vi "2048.vi"() -> ()   [LabVIEW 2013]
uses:
  <vilib>/Utility/file.llb/Read From Spreadsheet File (DBL).vi
  <vilib>/Utility/file.llb/Write To Spreadsheet File (I64).vi
panel:
  out "分数":i64=3
  in  "清空按钮":bool
  in  "按钮（退出程序）":bool
  out "错误输出":errorcluster
  in  "错误输入":errorcluster caption="错误输入（无错误）"
  out "2048":u16[][](array[ring])
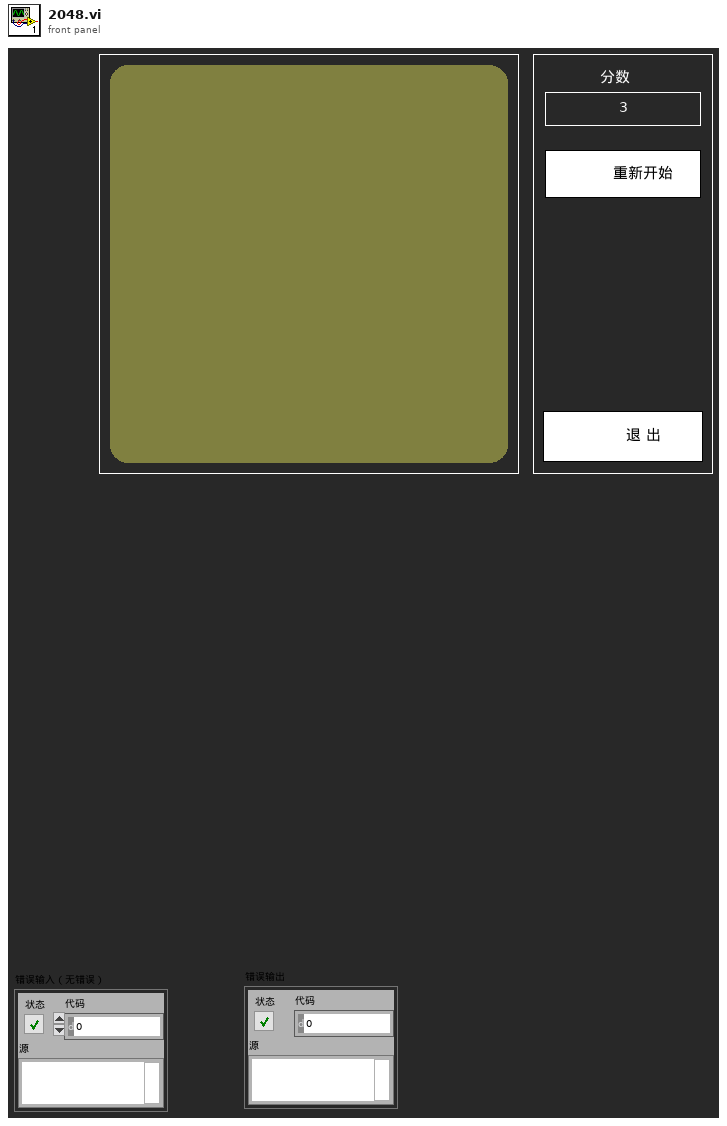
[diagram p1: front panel]
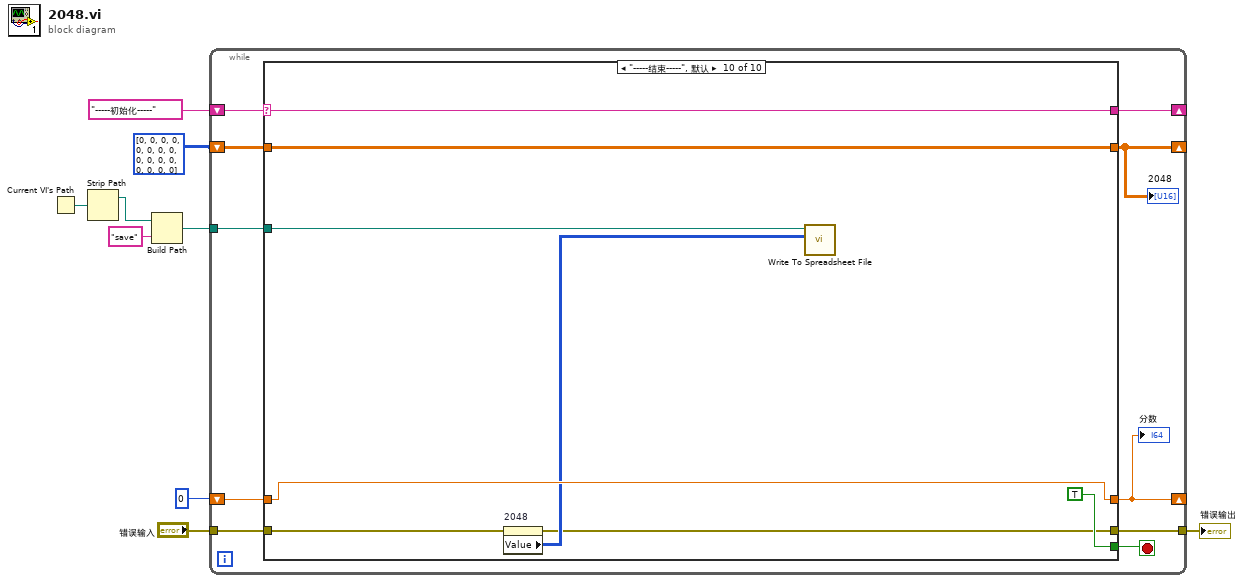
[diagram p0: block diagram]
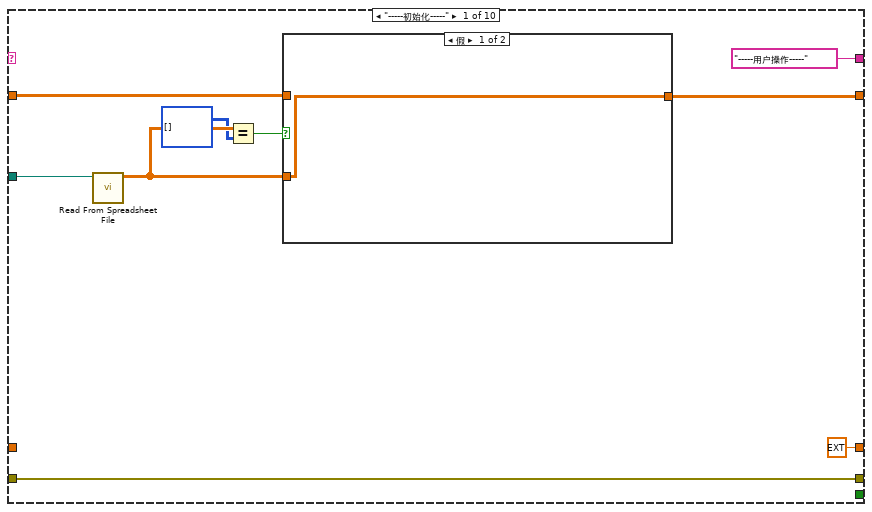
[diagram p2: hidden frame]
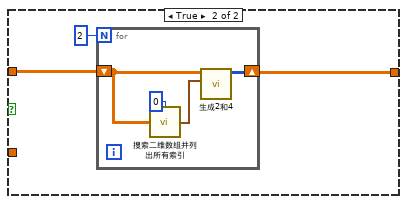
[diagram p3: hidden frame]
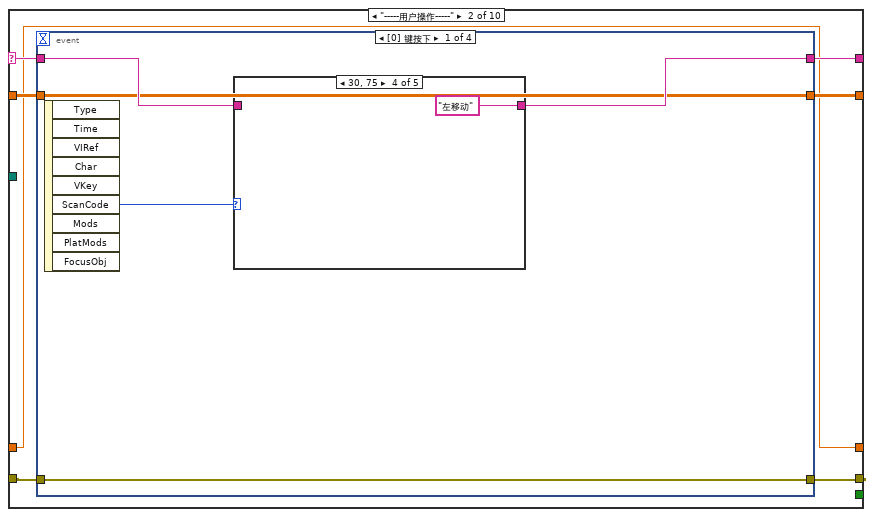
[diagram p4: hidden frame]
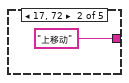
[diagram p6: hidden frame]
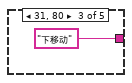
[diagram p7: hidden frame]
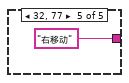
[diagram p8: hidden frame]
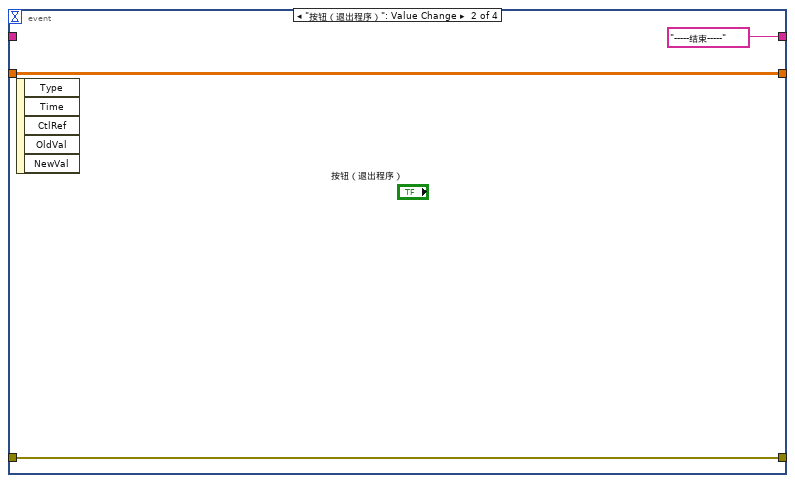
[diagram p9: hidden frame]
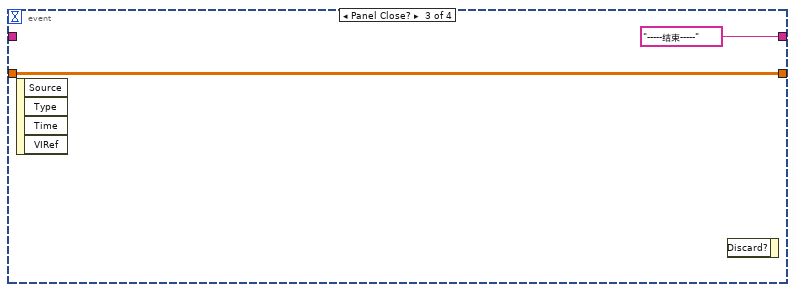
[diagram p10: hidden frame]
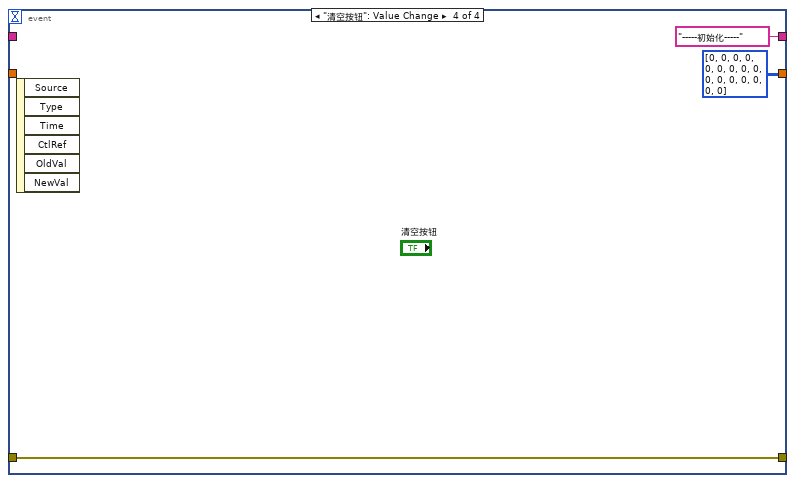
[diagram p11: hidden frame]
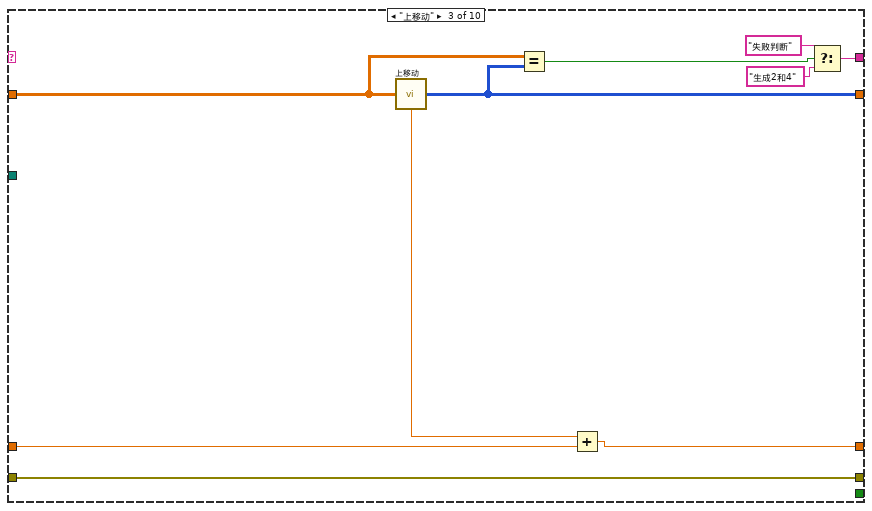
[diagram p12: hidden frame]
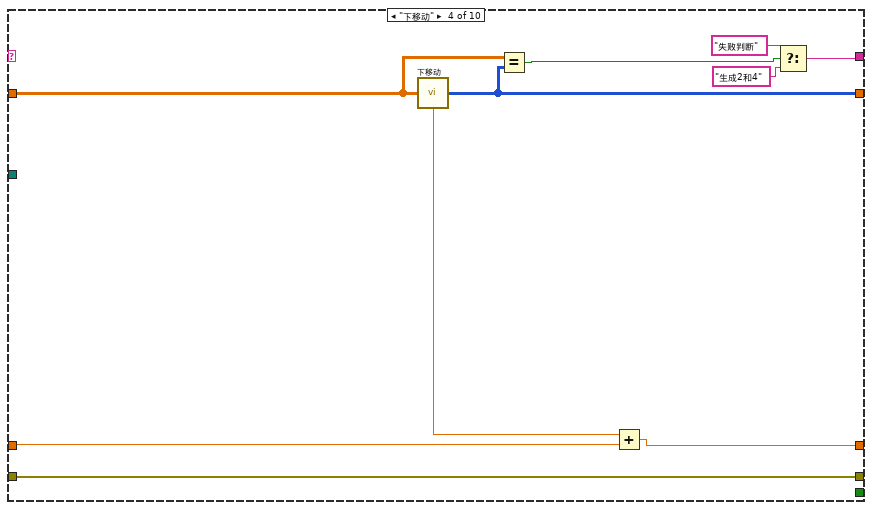
[diagram p13: hidden frame]
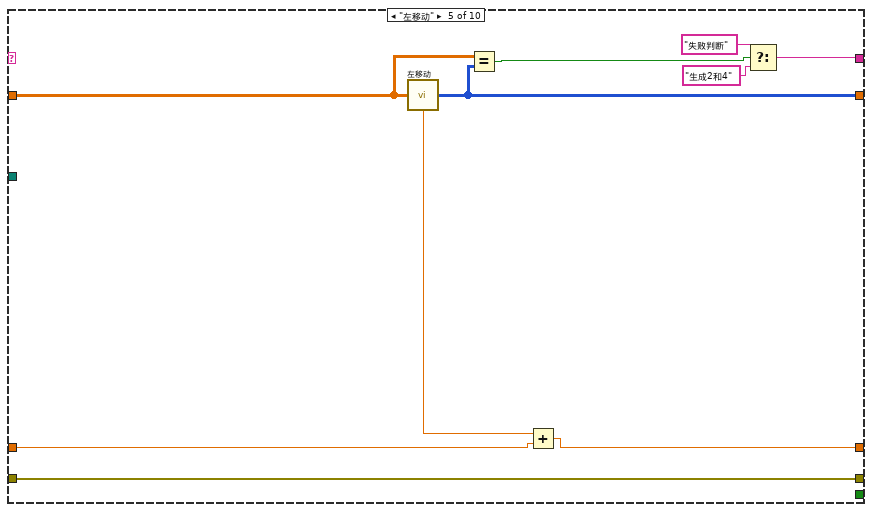
[diagram p14: hidden frame]
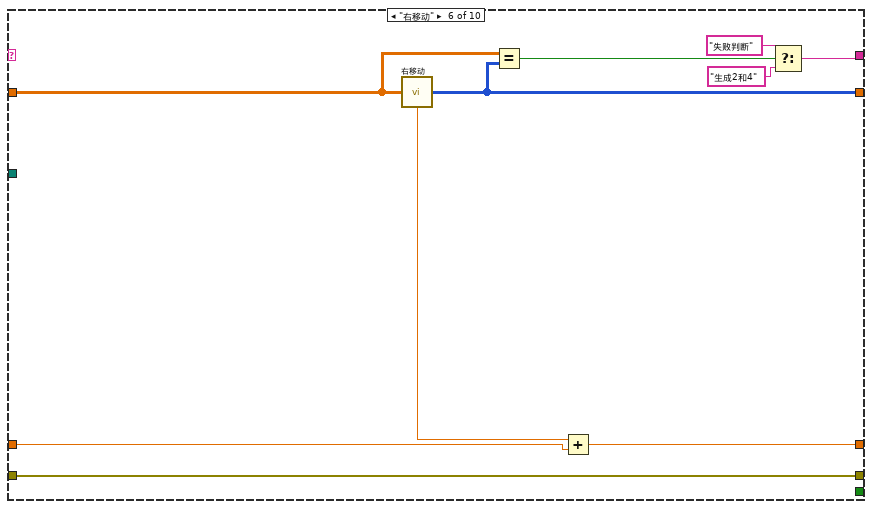
[diagram p15: hidden frame]
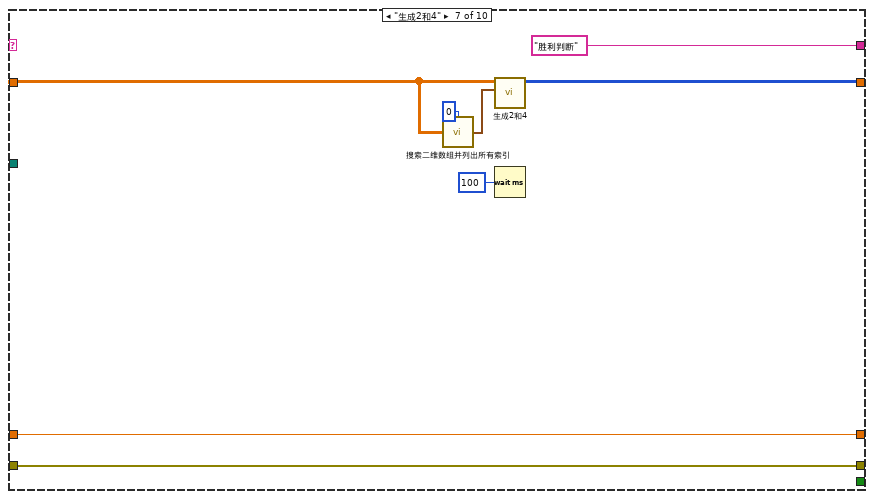
[diagram p16: hidden frame]
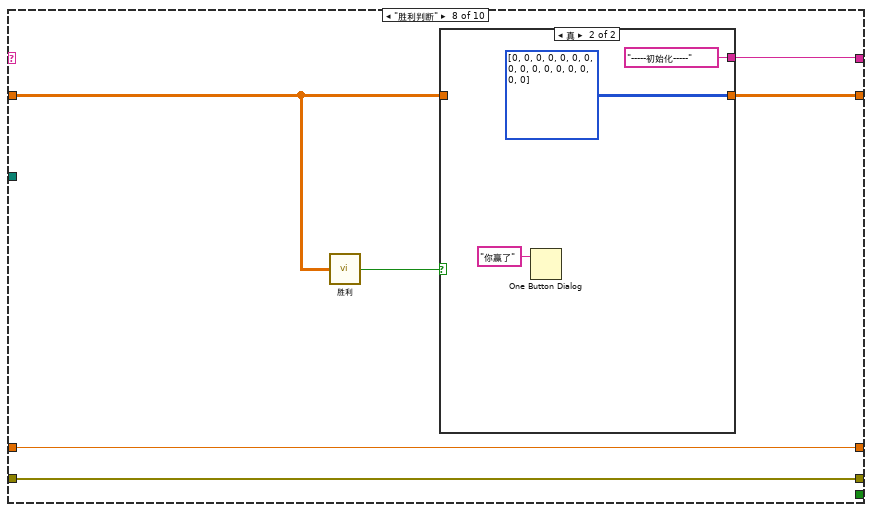
[diagram p17: hidden frame]
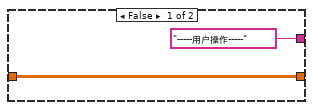
[diagram p18: hidden frame]
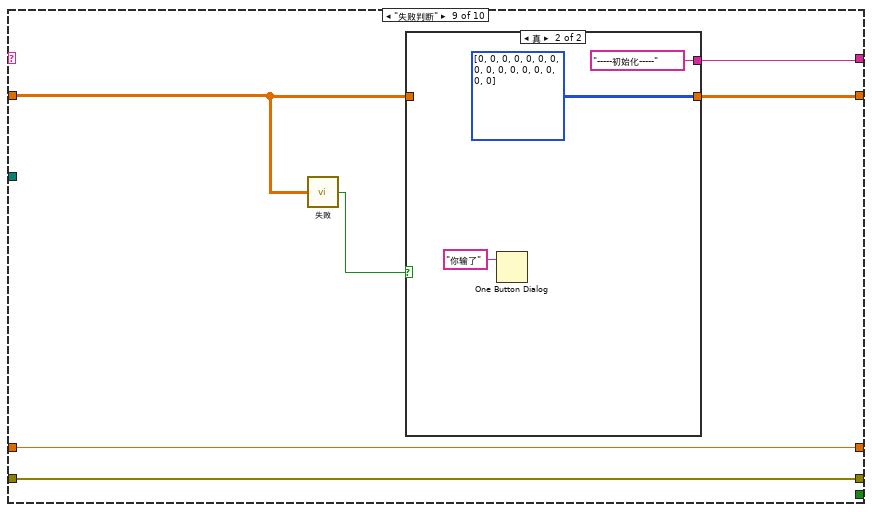
[diagram p19: hidden frame]
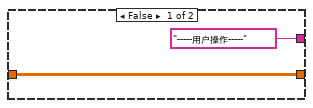
[diagram p20: hidden frame]
diagram:
  n1 = Current VI's Path() -> (path=w4:path)
  n2 = Strip Path(path=w4) -> (stripped path=w3:path)  [unwired: 1 out]
  n3 = Build Path(base path=w3, name or relative path="save" ("名称或相对路径")) -> (appended path=w1:path)
  n4 = while {
    shift-right: [w16] -> _
    shift-left: "-----初始化-----" -> [w17]
    tunnel: [w19] -> w8
    tunnel: "错误输入" -> [w18]
    shift-right: [w13] -> _
    shift-left: i32[][] [[0, 0, 0, 0], [0, 0, 0, 0], [0, 0, 0, 0], [0, 0, 0, 0]] ("2048") -> [w14]
    shift-right: [w11] -> _
    shift-left: 0 -> [w12]
    tunnel: w1 -> [w10]
    stop <- w15 stop-if-true
    n5 = case shown="\"-----结束-----\", 默认" w17 {
      selector: w17 -> [_ w40 _ _ _ _ _ _ _ w139]
      tunnel: [w23 w43 w71 w81 w91 w101 w109 w115 w126 w132] -> w19
      tunnel: w18 -> [w23 w42 w71 w81 w91 w101 w109 w115 w126 w133]
      tunnel: ["-----用户操作-----" w41 w68 w77 w87 w97 "胜利判断" w111 w125 w139] -> w16
      tunnel: [_ _ _ _ _ _ _ _ _ TRUE] -> w15
      tunnel: [w26 w39 w66 w76 w86 w96 w106 w113 w124 w137] -> w13
      tunnel: w14 -> [w27 w38 w67 w75 w85 w95 w105 w112 w123 w137]
      tunnel: w12 -> [_ w37 w63 w73 w83 w93 w102 w110 w121 w136]
      tunnel: [ext 0.0 w37 w62 w74 w82 w94 w102 w110 w121 w136] -> w11
      tunnel: w10 -> [w24 _ _ _ _ _ _ _ _ w135]
      frame "-----初始化-----" {
        n6 = call-poly <vilib>:"Read From Spreadsheet File.vi"("file path (dialog if empty)"=w24) -> ("all rows"=w21:dbl[][])  [unwired: 6 in, 4 out]
        n7 = Equal?(x=w21, y=i32[][] [] ("2048")) -> (x = y?=w22:bool)
        n8 = case shown="假" w22 {
          tunnel: w27 -> [_ w32]
          tunnel: [w29 w31] -> w26
          tunnel: w21 -> [w29 _]
          frame False {
          }
          frame True {
            n9 = for {
              N: 2 -> [_]
              shift-right: [w33] -> w31
              shift-left: w32 -> [w35]
              n10 = call "搜索二维数组并列出所有索引.vi"("搜索值"=0, "数组"=w35) -> ("索引数组"=w34:cluster{i32, i32}[])  [unwired: 2 in]
              n11 = call "生成2和4.vi"("索引数组"=w34, "2048输入"=w35) -> ("2048输出"=w33:i32[][])  [unwired: 9 in]
            }
          }
        }
      }
      frame "-----用户操作-----" {
        n12 = event shown="[0] 键按下" {
          selector: _ -> [_ _ _ _]
          dyn-events: _ -> [_ _ _ _]
          timeout: _ -> [_ _ _ _]
          tunnel: [w48 w56 _ w61] -> w43
          tunnel: w42 -> [w48 w56 _ w61]
          tunnel: [w47 "-----结束-----" "-----结束-----" "-----初始化-----"] -> w41
          tunnel: w40 -> [w46 _ _ _]
          tunnel: [w44 w54 w57 i32[][] [[0, 0, 0, 0], [0, 0, 0, 0], [0, 0, 0, 0], [0, 0, 0, 0]] ("2048")] -> w39
          tunnel: w38 -> [w44 w54 w57 _]
          event Key Down {
            n13 = event-data() -> ("ScanCode"=w45:i16)  [unwired: 1 in, 8 out]
            n14 = case shown="30, 75" w45 {
              tunnel: [w49 "上移动" "下移动" "左移动" "右移动"] -> w47
              tunnel: w46 -> [w49 _ _ _ _]
              frame 0, Default {
              }
              frame 17, 72 {
              }
              frame 31, 80 {
              }
              frame 30, 75 {
              }
              frame 32, 77 {
              }
            }
          }
          event "按钮（退出程序）": Value Change {
            n15 = event-data() -> ()  [unwired: 1 in, 5 out]
          }
          event Panel Close? {
            n16 = event-data() -> ()  [unwired: 1 in, 4 out]
            n17 = event-data() -> ()  [unwired: 2 in, 1 out]
          }
          event "清空按钮": Value Change {
            n18 = event-data() -> ()  [unwired: 1 in, 6 out]
          }
        }
      }
      frame "上移动" {
        n19 = call "上移动.vi"("移动前"=w67) -> ("移动后"=w66:i32[][], "分数"=w64:ext)  [unwired: 2 in]
        n20 = Equal?(x=w67, y=w66) -> (x = y?=w65:bool)
        n21 = Add(x=w64, y=w63) -> (x+y=w62:ext)
        n22 = Select(t="失败判断", s=w65, f="生成2和4") -> (s? t:f=w68:string)
      }
      frame "下移动" {
        n23 = call "下移动.vi"("移动前"=w75) -> ("移动后"=w76:i32[][], "分数"=w72:ext)  [unwired: 2 in]
        n24 = Equal?(x=w75, y=w76) -> (x = y?=w78:bool)
        n25 = Add(x=w72, y=w73) -> (x+y=w74:ext)
        n26 = Select(t="失败判断", s=w78, f="生成2和4") -> (s? t:f=w77:string)
      }
      frame "左移动" {
        n27 = call "左移动.vi"("移动前"=w85) -> ("移动后"=w86:i32[][], "分数"=w84:ext)  [unwired: 2 in]
        n28 = Equal?(x=w85, y=w86) -> (x = y?=w88:bool)
        n29 = Add(x=w84, y=w83) -> (x+y=w82:ext)
        n30 = Select(t="失败判断", s=w88, f="生成2和4") -> (s? t:f=w87:string)
      }
      frame "右移动" {
        n31 = call "右移动.vi"("移动前"=w95) -> ("移动后"=w96:i32[][], "分数"=w92:ext)  [unwired: 2 in]
        n32 = Equal?(x=w95, y=w96) -> (x = y?=w98:bool)
        n33 = Add(x=w92, y=w93) -> (x+y=w94:ext)
        n34 = Select(t="失败判断", s=w98, f="生成2和4") -> (s? t:f=w97:string)
      }
      frame "生成2和4" {
        n35 = call "搜索二维数组并列出所有索引.vi"("搜索值"=0, "数组"=w105) -> ("索引数组"=w108:cluster{i32, i32}[])  [unwired: 2 in]
        n36 = call "生成2和4.vi"("索引数组"=w108, "2048输入"=w105) -> ("2048输出"=w106:i32[][])  [unwired: 9 in]
        n37 = Wait (ms)(milliseconds to wait=u32 100 ("等待时间（毫秒）")) -> ()  [unwired: 1 out]
      }
      frame "胜利判断" {
        n38 = call "胜利.vi"("移动前"=w112) -> ("胜利？"=w114:bool)
        n39 = case shown="真" w114 {
          tunnel: [w117 i32[][] [[0, 0, 0, 0], [0, 0, 0, 0], [0, 0, 0, 0], [0, 0, 0, 0]] ("2048")] -> w113
          tunnel: w112 -> [w117 _]
          tunnel: ["-----用户操作-----" "-----初始化-----"] -> w111
          frame False {
          }
          frame True {
            n40 = One Button Dialog(message="你赢了" ("消息")) -> ()  [unwired: 1 in, 1 out]
          }
        }
      }
      frame "失败判断" {
        n41 = call "失败.vi"("移动前"=w123) -> ("失败？"=w122:bool)
        n42 = case shown="真" w122 {
          tunnel: ["-----用户操作-----" "-----初始化-----"] -> w125
          tunnel: [w127 i32[][] [[0, 0, 0, 0], [0, 0, 0, 0], [0, 0, 0, 0], [0, 0, 0, 0]] ("2048")] -> w124
          tunnel: w123 -> [w127 _]
          frame False {
          }
          frame True {
            n43 = One Button Dialog(message="你输了" ("消息")) -> ()  [unwired: 1 in, 1 out]
          }
        }
      }
      frame "-----结束-----", Default {
        n44 = property on="2048" class="Arr (严格)"(error in=w133) -> (error out=w132:errorcluster, "Value"=w134:u16[][])  [unwired: 1 in, 1 out]
        n45 = call-poly <vilib>:"Write To Spreadsheet File.vi"("2D data"=w134, "file path (dialog if empty)"=w135) -> ()  [unwired: 6 in, 1 out]
      }
    }
    "2048" <- w13
    "分数" <- w11
  }
  "错误输出" <- w8
